vi "GlobalFavoriteNames.vi"() -> ()   [LabVIEW 2015]
panel:
  in  "Favorite Names":string[](array[string])
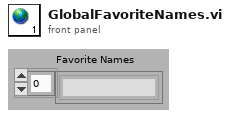
[diagram p1: front panel]
diagram:
